vi "AssertValueByArrayName.vi"(0 "VI Reference In":refnum<vi>, 1 "Test Label":string, 2 "delimiter (>>)":string=">>", 3 "Assert Only? (F)":bool, 5 "Control Path":string, 7 "Focus Item Names":string[](array[string]), 11 "Error In":errorcluster, 12 "Assert Interval(10 ms)":u32=10, 13 "Timeout(5 sec)":dbl=5.0) -> (4 "VI Reference Out":refnum<vi>, 6 "Asserted Value":string[](array[string]), 15 "Error Out":errorcluster)   [LabVIEW 2016, in "Drona.lvlib" / "AssertControlValue.lvlib" / "AssertListbox.lvlib"]
doc: "Asserts if the focus item names of multi-select listbox control are equal.\n\nThe input control name is given as a string , incase of path, use delimiters inbetween the path.\nThis VI gets the value of the control, untill the value is equal to the input value."
uses:
  AssertListbox.lvlib
  Get/GetControlRef/GetControlRefByPath.vi
  <userlib>/_OpenG.lib/array/array.llb/Index 1D Array Elements (String)__ogtk.vi
  <vilib>/addons/_JKI Toolkits/Caraya/classes/Assert/Assert Equal Value_Variant.vi
  <vilib>/Utility/error.llb/Error Cluster From Error Code.vi
  <vilib>/ErrorRing/Error Ring.xnode
  <vilib>/addons/_JKI Toolkits/Caraya/classes/Assert/Assert.lvclass
  Get/GetControlRef/GetControlRef.lvlib
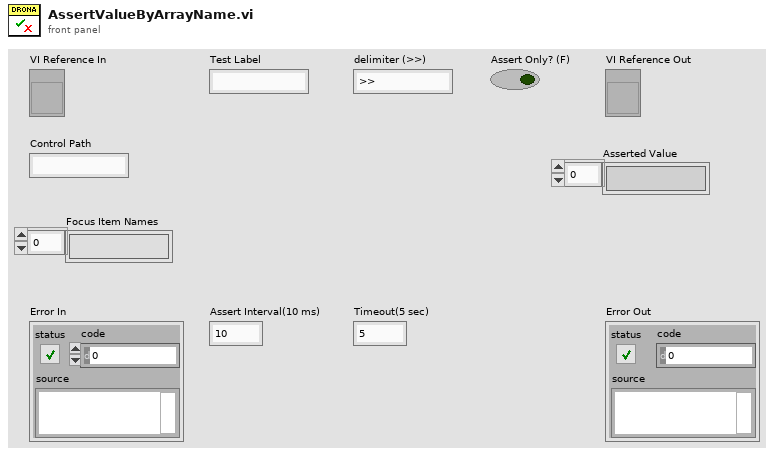
[diagram p1: front panel]
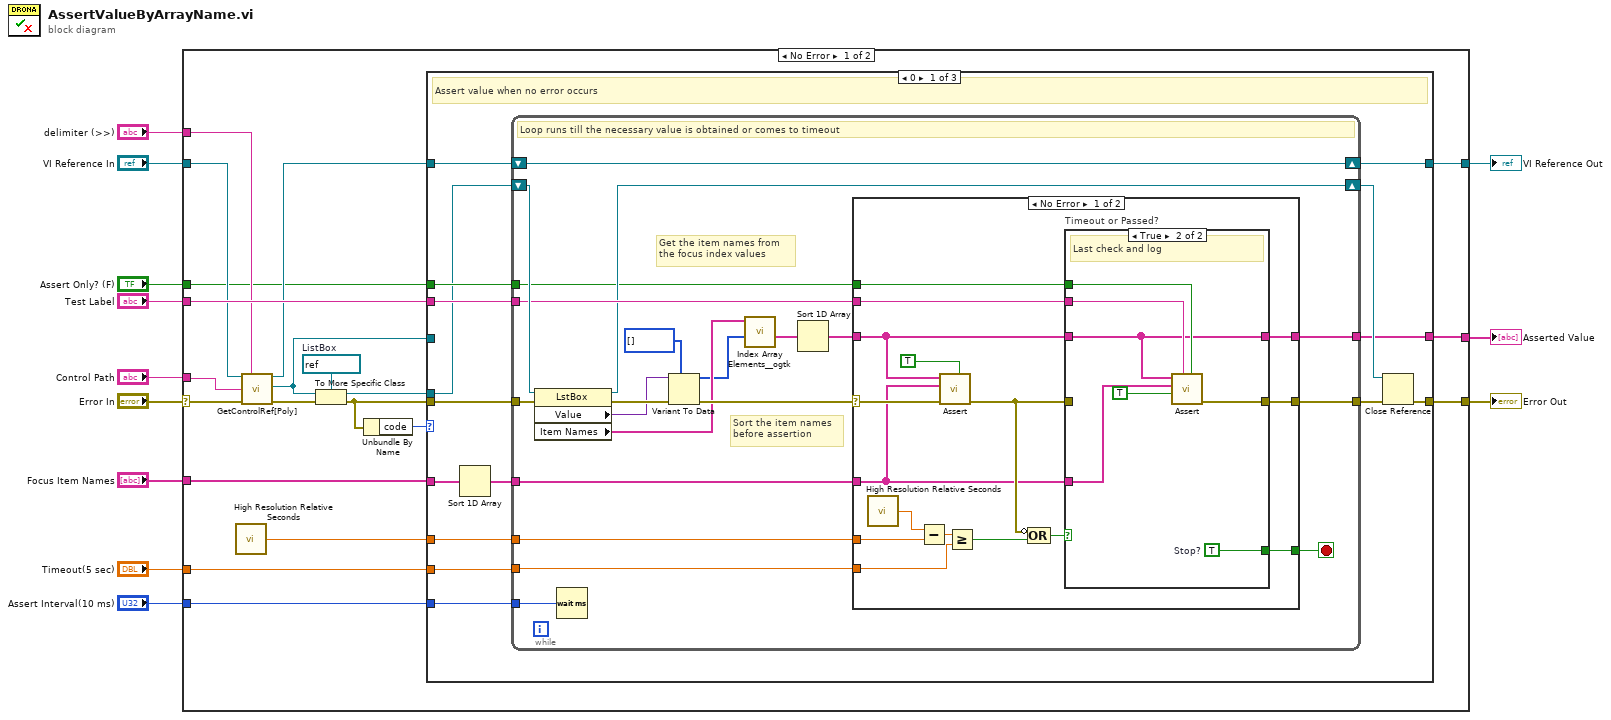
[diagram p0: block diagram]
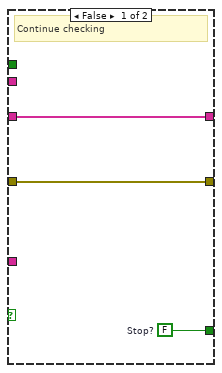
[diagram p2: hidden frame]
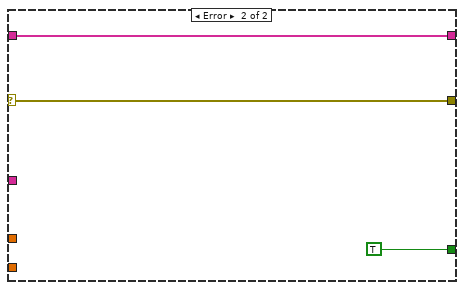
[diagram p3: hidden frame]
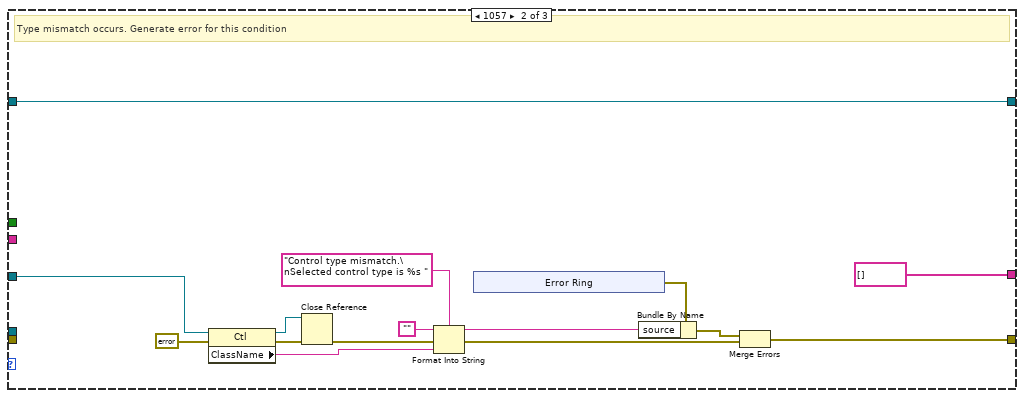
[diagram p4: hidden frame]
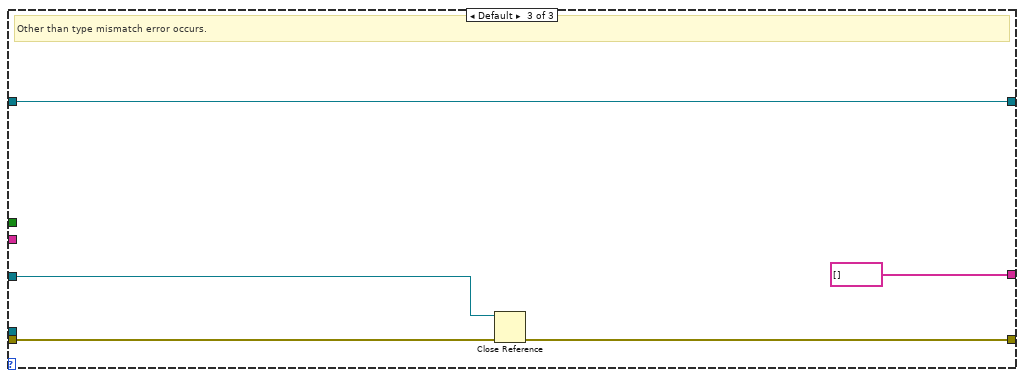
[diagram p5: hidden frame]
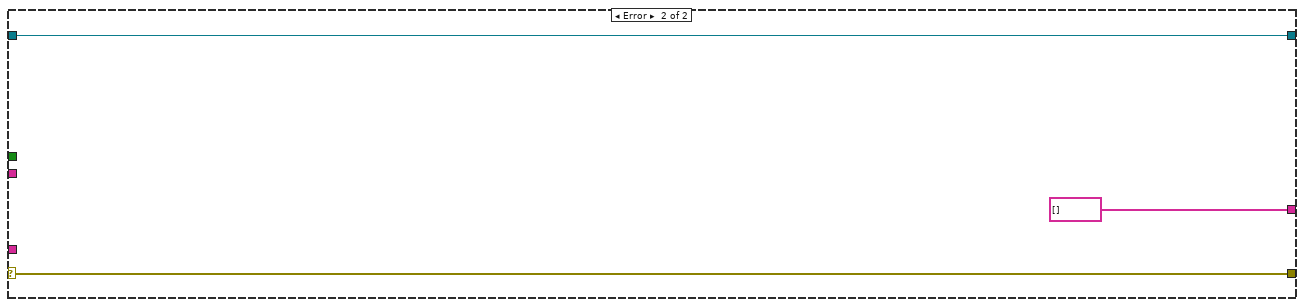
[diagram p6: hidden frame]
diagram:
  n1 = case shown="No Error" "Error In" {
    selector: "Error In" -> [w28 w125]
    tunnel: "Timeout(5 sec)" -> [w32 _]
    tunnel: [w31 w124] -> w11
    tunnel: [w22 w125] -> w10
    tunnel: "Assert Interval(10 ms)" -> [w30 _]
    tunnel: "Test Label" -> [w29 _]
    tunnel: "VI Reference In" -> [w27 w124]
    tunnel: "Control Path" -> [w26 _]
    tunnel: "delimiter (>>)" -> [w21 _]
    tunnel: "Assert Only? (F)" -> [w20 _]
    tunnel: [w19 string[] []] -> w2
    tunnel: "Focus Item Names" -> [w16 _]
    frame No Error {
      w18 = refnum<vi> refnum  # ListBox
      n2 = call <vilib>:"High Resolution Relative Seconds.vi"() -> ("relative seconds"=w25:dbl)
      n3 = call-poly "GetControlRef[Poly].vi"("VI Reference In"=w27, "delimiter (>>)"=w21, "Control Path"=w26, "error In"=w28) -> ("VI Reference Out"=w23:refnum<vi>, "Ctl Refnum"=w13:refnum<vi>, "error out"=w24:errorcluster)  [unwired: 9 in]
      n4 = To More Specific Class(target class=w18, reference=w13, error in=w24) -> (specific class reference=w17:refnum<vi>, error out=w15:errorcluster)
      n5 = Unbundle By Name(w15) -> ("code"=w14:i32)
      n6 = case shown="0" w14 {
        tunnel: w32 -> [w47 _ _]
        tunnel: [w46 w98 w121] -> w31
        tunnel: w30 -> [w44 _ _]
        tunnel: w29 -> [w43 _ _]
        tunnel: w25 -> [w42 _ _]
        tunnel: w23 -> [w41 w98 w121]
        tunnel: [w40 w101 w119] -> w22
        tunnel: w20 -> [w38 _ _]
        tunnel: [w33 string[] [] string[] []] -> w19
        tunnel: w15 -> [w37 _ w122]
        tunnel: w17 -> [w36 _ _]
        tunnel: w16 -> [w35 _ _]
        tunnel: w13 -> [_ w100 w118]
        frame 0 {
          # "Assert value when no error occurs"
          n7 = Sort 1D Array(array=w35) -> (sorted array=w34:string[])
          n8 = while {
            tunnel: w47 -> [w67]
            tunnel: w42 -> [w68]
            tunnel: w37 -> [w62]
            tunnel: [w65] -> w45
            tunnel: w44 -> [w63]
            tunnel: w43 -> [w59]
            shift-right: [w60] -> w46
            shift-left: w41 -> [w60]
            shift-right: [w58] -> w39
            shift-left: w36 -> [w61]
            tunnel: w38 -> [w57]
            tunnel: [w56] -> w33
            tunnel: w34 -> [w52]
            stop <- w66 stop-if-true
            # "Sort the item names \nbefore assertion"
            # "Get the item names from \nthe focus index values"
            # "Loop runs till the necessary value is obtained or comes to timeout"
            n9 = property on="Property Node" class="LstBox"(reference=w61, error in=w62) -> (reference out=w58:refnum<vi>, error out=w64:errorcluster, "Value"=w54:variant, "Item Names"=w50:string[])
            n10 = Wait (ms)(milliseconds to wait=w63) -> ()  [unwired: 1 out]
            n11 = Variant To Data(error in=w64, type=i32[] [], Variant=w54) -> (data=w49:i32[], error out=w55:errorcluster)
            n12 = call-poly <userlib>:"Index Array Elements__ogtk.vi"("indices"=w49, "array"=w50) -> ("elements"=w48:string[])  [unwired: 9 in]
            n13 = Sort 1D Array(array=w48) -> (sorted array=w51:string[])
            n14 = case shown="No Error" w55 {
              selector: w55 -> [w80 w97]
              tunnel: w68 -> [w84 _]
              tunnel: w67 -> [w81 _]
              tunnel: [w71 TRUE] -> w66
              tunnel: [w72 w97] -> w65
              tunnel: w52 -> [w73 _]
              tunnel: w51 -> [w74 w95]
              tunnel: w59 -> [w79 _]
              tunnel: w57 -> [w70 _]
              tunnel: [w69 w95] -> w56
              frame No Error {
                n15 = call <vilib>:"High Resolution Relative Seconds.vi"() -> ("relative seconds"=w83:dbl)
                n16 = Subtract(x=w83, y=w84) -> (x-y=w82:dbl)
                n17 = call-poly <vilib>:"Assert.vi"("Assert Only? (F)"=TRUE, "error in (no error)"=w80, "Y"=w73, "X"=w74) -> ("error out"=w77:errorcluster)  [unwired: 7 in]
                n18 = Greater Or Equal?(x=w82, y=w81) -> (x >= y?=w78:bool)
                n19 = Compound Arithmetic op=OR(invert w77, w78) -> (w76:bool)
                n20 = case "Timeout or Passed?" shown="True" w76 {
                  tunnel: w77 -> [w87 _]
                  tunnel: w73 -> [_ w89]
                  tunnel: w74 -> [w85 w90]
                  tunnel: w79 -> [_ w94]
                  tunnel: [w87 w93] -> w72
                  tunnel: [w86 w92] -> w71
                  tunnel: w70 -> [_ w91]
                  tunnel: [w85 w90] -> w69
                  frame False {
                    w86 = FALSE  # Stop?
                    # "Continue checking"
                  }
                  frame True {
                    w92 = TRUE  # Stop?
                    # "Last check and log"
                    n21 = call-poly <vilib>:"Assert.vi"("Assert Only? (F)"=w91, "Label"=w94, "Register with caller test (F)"=TRUE, "Y"=w89, "X"=w90) -> ("error out"=w93:errorcluster)  [unwired: 6 in]
                  }
                }
              }
              frame Error {
              }
            }
          }
          n22 = Close Reference(reference=w39, error in (no error)=w45) -> (error out=w40:errorcluster)
        }
        frame 1057 {
          # "Type mismatch occurs. Generate error for this condition"
          n23 = property class="Ctl"(reference=w100, error in=errorcluster {"status"=FALSE, "code"=0, "source"=""} ("error out")) -> (reference out=w102:refnum<vi>, error out=w112:errorcluster, "ClassName"=w109:string)
          n24 = Close Reference(reference=w102, error in (no error)=w112) -> (error out=w103:errorcluster)
          n25 = Format Into String(format string="Control type mismatch.\nSelected control type is %s ", initial string="", error in=w103, w109) -> (resulting string=w106:string, error out=w104:errorcluster)
          n26 = xnode "Error Ring"() -> ("error out"=w107:errorcluster)
          n27 = Bundle By Name(cluster=w107, "source"=w106) -> (w105:errorcluster)
          n28 = Merge Errors(w105, w104) -> (w101:errorcluster)
        }
        frame Default {
          # "Other than type mismatch error occurs."
          n29 = Close Reference(reference=w118, error in (no error)=w122) -> (error out=w119:errorcluster)
        }
      }
    }
    frame Error {
    }
  }
  "Error Out" <- w10
  "VI Reference Out" <- w11
  "Asserted Value" <- w2
